vi "Do Core.vi"(8 "error in (no error)":errorcluster, 9 "Actor in":refnum<class "Actor.lvclass">, 11 "Reply Message":refnum<class "Read Sample from Container Msg.lvclass">) -> (0 "error out":errorcluster, 1 "Actor out":refnum<class "Actor.lvclass">, 2 "Reply":variant)   [LabVIEW 2015, in "cRIO-Carbondioxide.lvlib" / "CO2-Actor.lvlib" / "Read Sample from Container Msg.lvclass"]
doc: "(<B>Filename</B>: Actor Framework.lvlib:Reply Msg.lvclass:Do Core.vi)\n\nDefines what an actor does when it receives <B>Reply Message</B>. This method also defines the <B>Reply</B> that is returned to the actor that sent <B>Reply Message</B>.\n\nBy default, this method does nothing, and <B>Reply</B> is the ancestor Message class. A child class must override this method to define behavior and specify a child of the Message class to return in the <B>Reply</B> output."
uses:
  Read Sample from Container Msg.lvclass
  <vilib>/ActorFramework/Actor/Actor.lvclass
  Read Sample from Container Msg.lvclass/Read Sample from Container Msg.ctl
  CO2 Actor/CO2 Actor.lvclass
  <vilib>/ActorFramework/Reply Msg/Reply Msg.lvclass
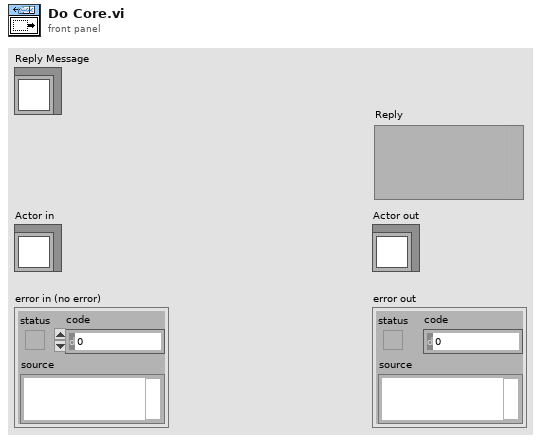
[diagram p1: front panel]
types:
  T1 = typedef "Sample Transfer Container Enumerator.ctl" = enum16{"None", "Sample 1", "Sample 2", "Sample 3", "Sample 4", "Sample 5", "Storage 01", "Storage 02", "Storage 03", "Storage 04", "Storage 05", "Storage 06", "Storage 07", "Storage 08", "Storage 09", "Storage 10", "Storage 11", "Storage 12", "Syringe", "Undefined"}
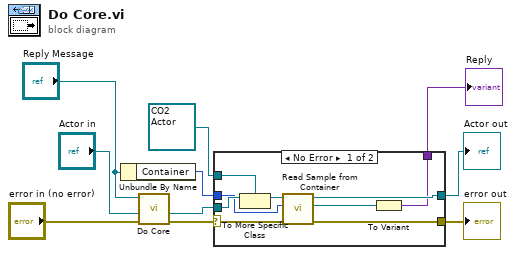
[diagram p0: block diagram]
diagram:
  n1 = Unbundle By Name("Reply Message") -> ("Container"=w2:T1)
  n2 = call-parent "Do Core.vi"("error in (no error)"="error in (no error)", "Actor in"="Actor in", "Reply Message"="Reply Message") -> ("error out"=w7:errorcluster, "Actor out"=w4:refnum<class "Actor.lvclass">)  [unwired: 6 in, 1 out]
  n3 = case shown="No Error" w7 {
    selector: w7 -> [w17 w21]
    tunnel: [w19 w21] -> w6
    tunnel: [w18 w20] -> w5
    tunnel: w4 -> [w16 w20]
    tunnel: refnum<class "CO2 Actor.lvclass"> refnum ("CO2 Actor in") -> [w15 _]
    tunnel: w2 -> [w13 _]
    tunnel: [w11 _] -> w1
    frame No Error {
      n4 = To More Specific Class(target class=w15, reference=w16) -> (specific class reference=w14:refnum<class "CO2 Actor.lvclass">)  [unwired: 1 in, 1 out]
      n5 = call-dynamic "Read Sample from Container.vi"("error in (no error)"=w17, "Container"=w13, "CO2 Actor in"=w14) -> ("error out"=w19:errorcluster, "Sample"=w12:refnum<class "Sample.lvclass">, "CO2 Actor out"=w18:refnum<class "CO2 Actor.lvclass">)  [unwired: 6 in]
      n6 = To Variant(anything=w12) -> (Variant=w11:variant)
    }
    frame Error {
      # "If type check fails, pass the original object out again."
    }
  }
  "error out" <- w6
  "Actor out" <- w5
  "Reply" <- w1
